vi "HCOP_FILE.vi"(0 "VISA IN":refnum<visa-resource-name>, 5 "error in":errorcluster, 7 "FileName":string) -> (14 "VISA Out":refnum<visa-resource-name>, 19 "error out":errorcluster)   [LabVIEW 2018, in "PNA-X.lvlib"]
doc: "HCOPy:FILE <filename> \n(Write-only) Saves the screen image to a file. \nParameters \n<filename> Name of the file to save the screen to. The file is saved to the current working \ndirectory unless a valid full path name is specified. \nUse one of the following suffixes: \n.bmp - not recommended due to large file size \n.jpg - not recommended due to poor quality \n.png - recommended \nExamples HCOPY:FILE \"myFile.png\" \nhcopy:file \"c:\\data\\myfile.png\" \nQuery Syntax Not Applicable \nDefault Not Applicable \nHCOPy[:IMMediate] \n(Write-only) Prints the screen to the default printer. \nExamples HCOP \nhcopy:immediate \nQuery Syntax Not applicable \nDefault Not Applicable \n1604\n\nInitiate Commands \nControls triggering signals \nClick on a blue keyword to view the command details. \nSee Also"
uses:
  PNA-X.lvlib
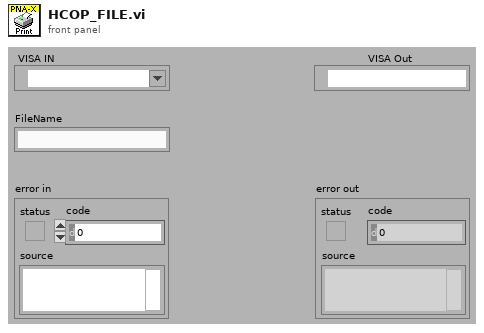
[diagram p1: front panel]
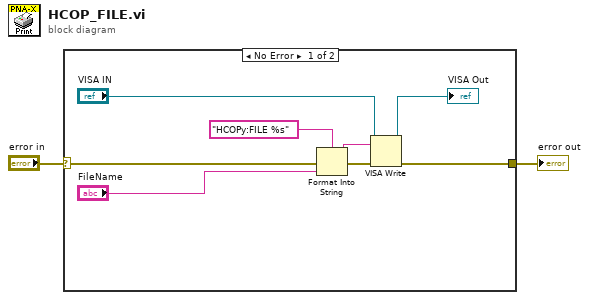
[diagram p0: block diagram]
diagram:
  n1 = case shown="No Error" "error in" {
    selector: "error in" -> [w10 w11]
    tunnel: [w5 w11] -> w1
    frame No Error {
      n2 = Format Into String(format string="HCOPy:FILE %s" ("Cmdline"), error in=w10, "FileName") -> (resulting string=w8:string, error out=w9:errorcluster)  [unwired: 1 in]
      n3 = VISA Write(VISA resource name="VISA IN", write buffer=w8, error in (no error)=w9) -> (VISA resource name out=→"VISA Out":refnum<visa-resource-name>, error out=w5:errorcluster)  [unwired: 1 out]
    }
    frame Error {
    }
  }
  "error out" <- w1
